vi "configuration UI.vi"() -> ()   [LabVIEW 2013, in "fixed channel editor.lvclass"]
uses:
  fixed channel editor.lvclass
  <vilib>/CEF_TreeControl/Node/NodeRef.ctl
  <vilib>/CEF_TreeControl/Node/NISE_CEF_Node.lvclass
  <vilib>/NI/AMC/Message Queue.ctl
  <vilib>/NI/AMC/Message.ctl
  <vilib>/NI/Tools/Keyed Array/KeyedArray.ctl
  <vilib>/CEF_TreeControl/Node/UserEventRef.ctl
  <vilib>/CEF_TreeControl/Controls/EventCluster.ctl
  <vilib>/NI/Tag Bus Module Framework/root configuration/TBM configuration.lvclass/TBM configuration.ctl
  <vilib>/NI/Tag Bus Module Framework/module configuration/TBM module configuration.lvclass
  <vilib>/NI/Tag Bus Module Framework/channel/TBM channel.lvclass
  <vilib>/NI/Tag Bus/tag/tag descriptor.lvclass/tag descriptor.ctl
  <vilib>/NI/Tag Bus Module Framework/channel/channel classification.ctl
  module/configuration/fixed channel configuration.lvclass
  <vilib>/NI/Tag Bus Module Framework/root configuration/Read instance name.vi
  read fixed channel configuration.vi
  <vilib>/NI/Tag Bus Module Framework/root configuration/create GUID.vi
  <vilib>/NI/Tag Bus Data Framework/Configuration Editor/Classes/Module editor node/Read Module Configuration.vi
  <vilib>/NI/Module Execution Interface/Engine Configuration/engine configuration.lvclass
  <vilib>/NI/Tag Bus/tag/tag descriptor.lvclass
  <vilib>/CEF_TreeControl/NISE_CEF_TreeControl.lvlib
  <vilib>/NI/Tag Bus Data Framework/Configuration Editor/Classes/Engine Parent/Engine Parent Editor Node.lvclass
  <vilib>/NI/Tag Bus Data Framework/Configuration Editor/Classes/Module editor node/module editor node.lvclass
  <vilib>/NI/Tools/Keyed Array/Tools_KeyedArray.lvlib
  <vilib>/NI/AMC/AMC.lvlib
panel:
  in  "Tab Control":enum32{"Channels", "Parameters"}(tab)
  in  "mapwriters":bool
  out "Channel List":string[][](table)
  in  "mapall":bool
  in  "kvp":i32(listbox)
  in  "user event":T1
  in  "main queue":T2
  in  "node ref":T3
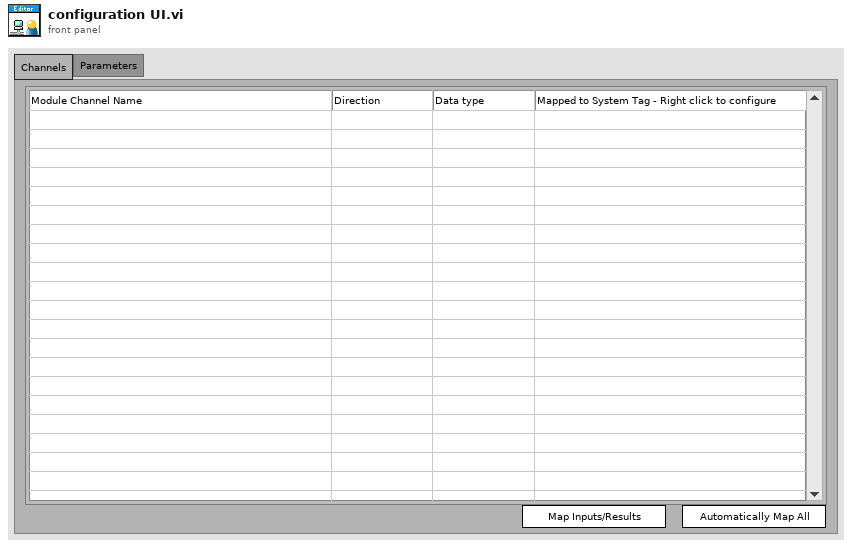
[diagram p1: front panel]
types:
  T1 = typedef "NISE_CEF_Node.lvclass/UserEventRef.ctl" = refnum<user-event>
  T2 = typedef "AMC.lvlib/Message Queue.ctl" = refnum<queue>
  T3 = typedef "NISE_CEF_Node.lvclass/NodeRef.ctl" = refnum<data-value>
  T4 = typedef "NISE_CEF_TreeControl.lvlib/EventCluster.ctl" = cluster{"command":string, "data":string}
  T5 = typedef "LVPoint32TypeDef.ctl" = cluster{"Horizontal":i32, "Vertical":i32}
  T6 = typedef "LVRowAndColumnTypeDef.ctl" = cluster{"Row":i32, "Column":i32}
  T7 = typedef "TBM channel.lvclass/channel classification.ctl" = enum16{"input data", "output data", "processing parameter", "processing result"}
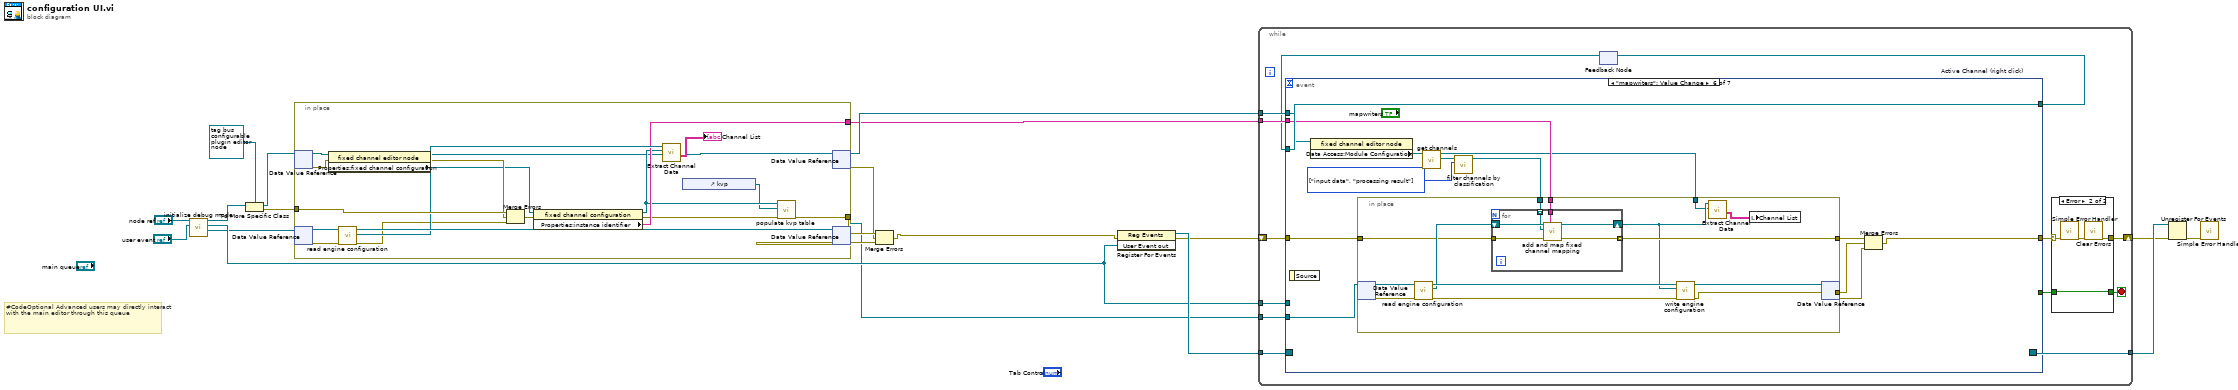
[diagram p0: block diagram]
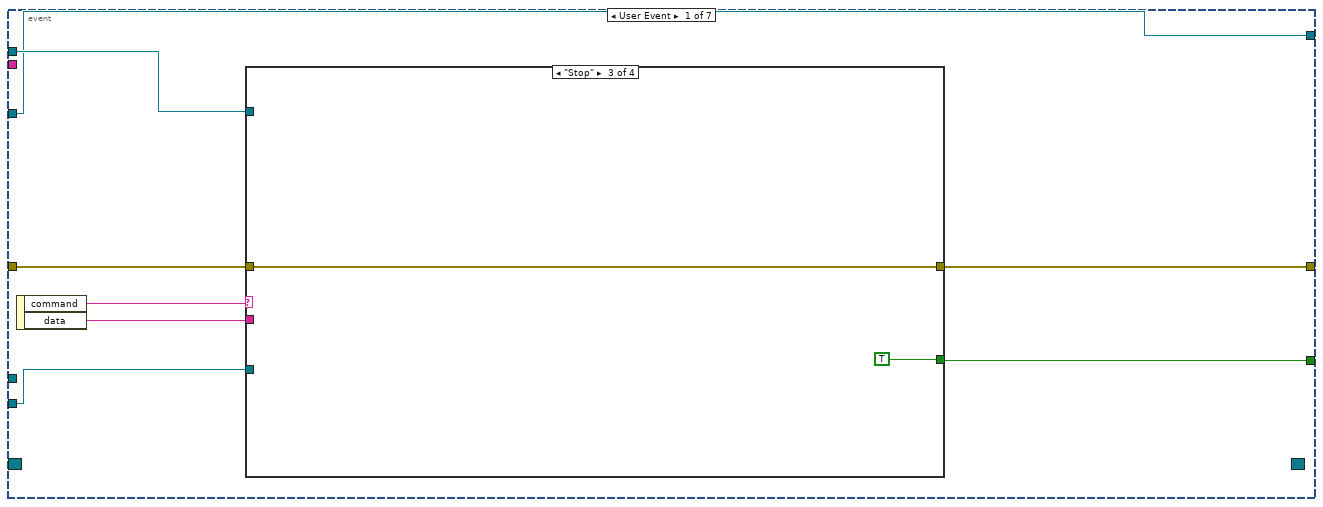
[diagram p3: hidden frame]
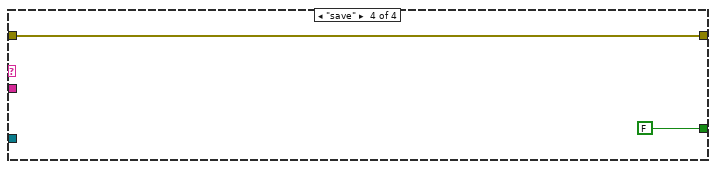
[diagram p6: hidden frame]
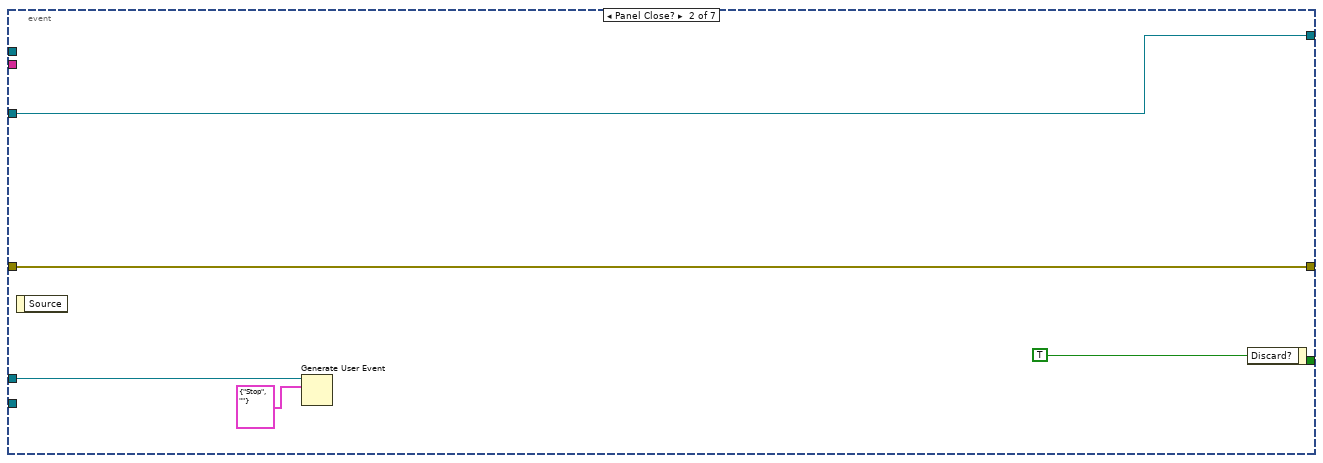
[diagram p7: hidden frame]
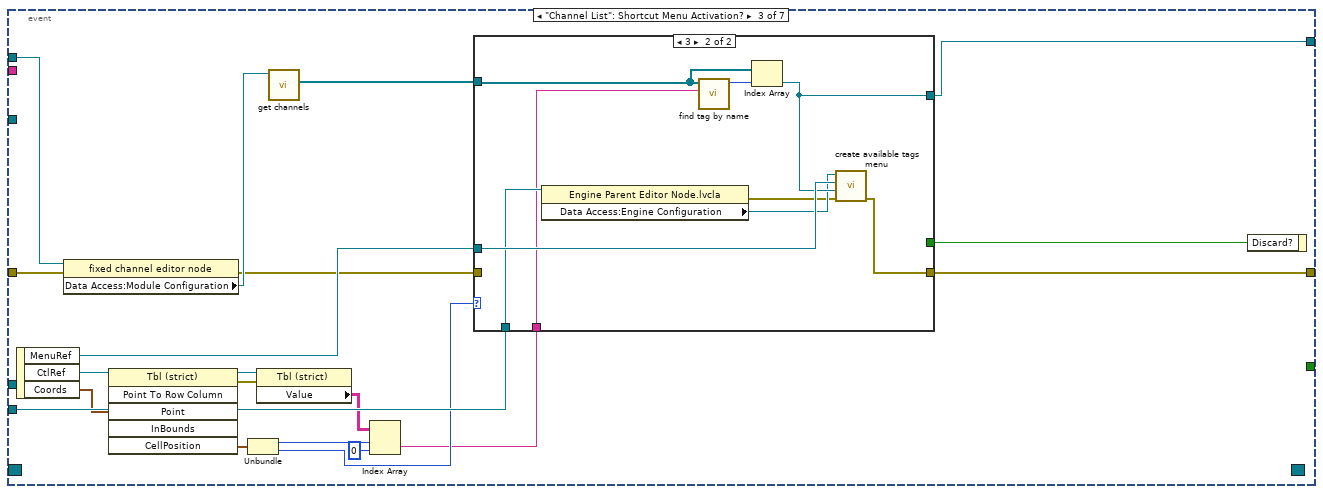
[diagram p8: hidden frame]
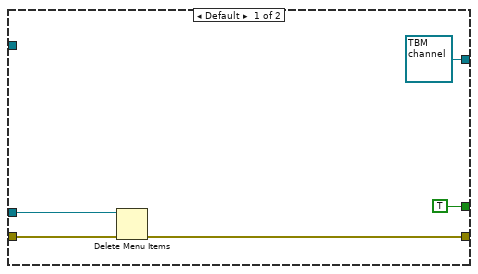
[diagram p9: hidden frame]
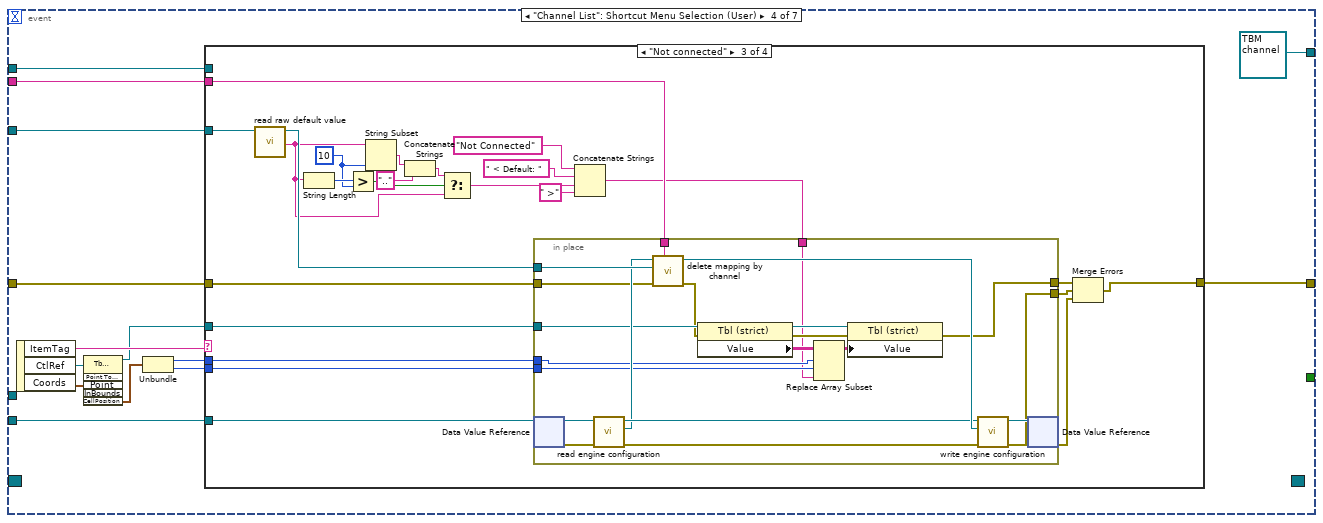
[diagram p10: hidden frame]
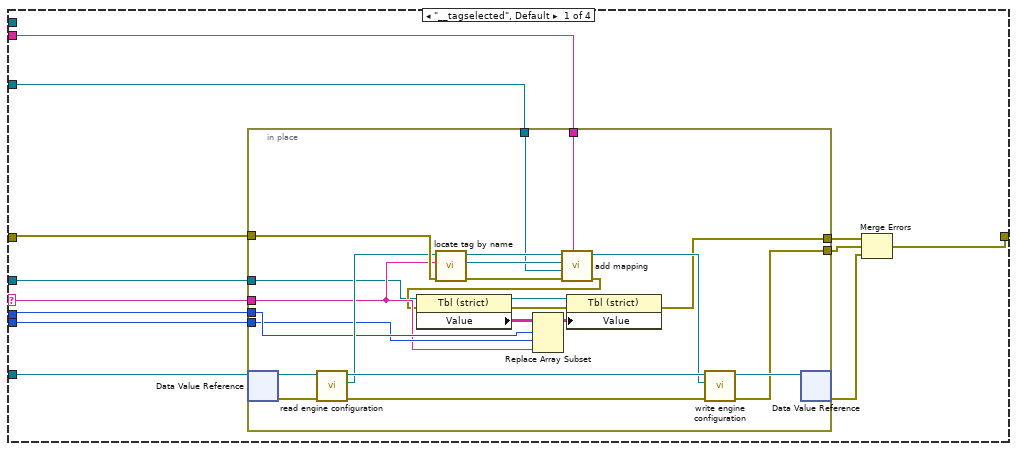
[diagram p11: hidden frame]
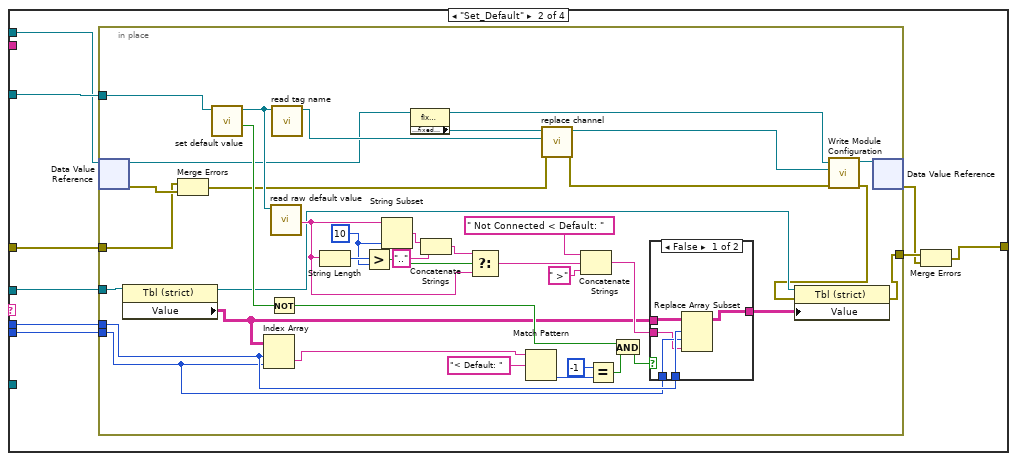
[diagram p12: hidden frame]
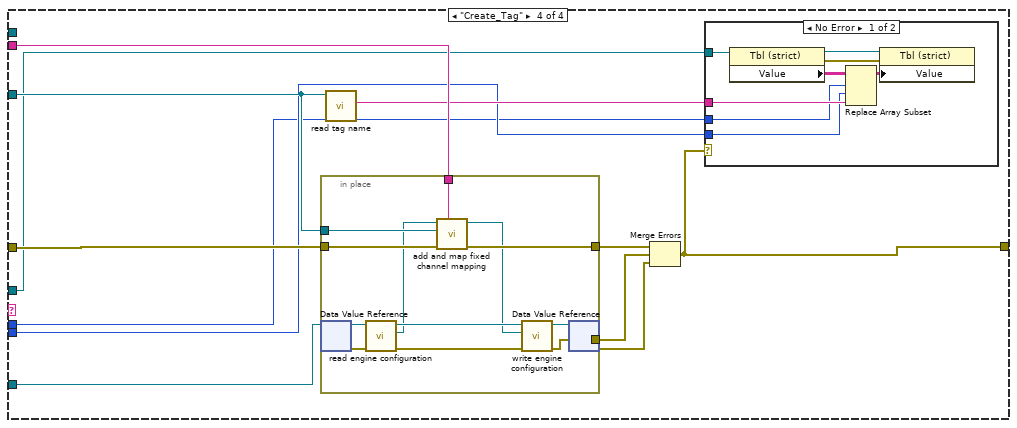
[diagram p14: hidden frame]
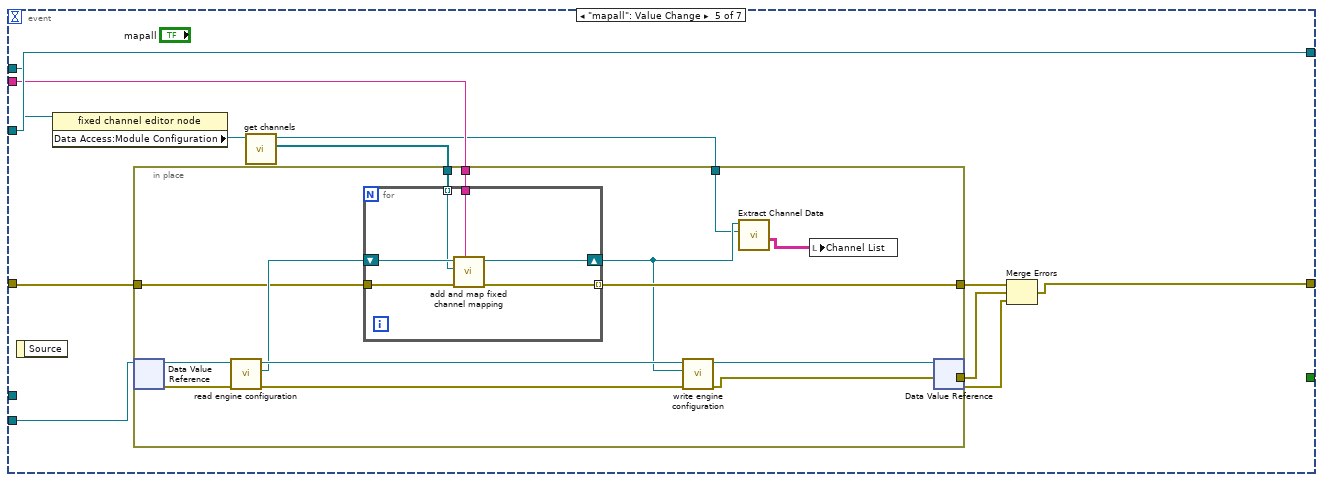
[diagram p16: hidden frame]
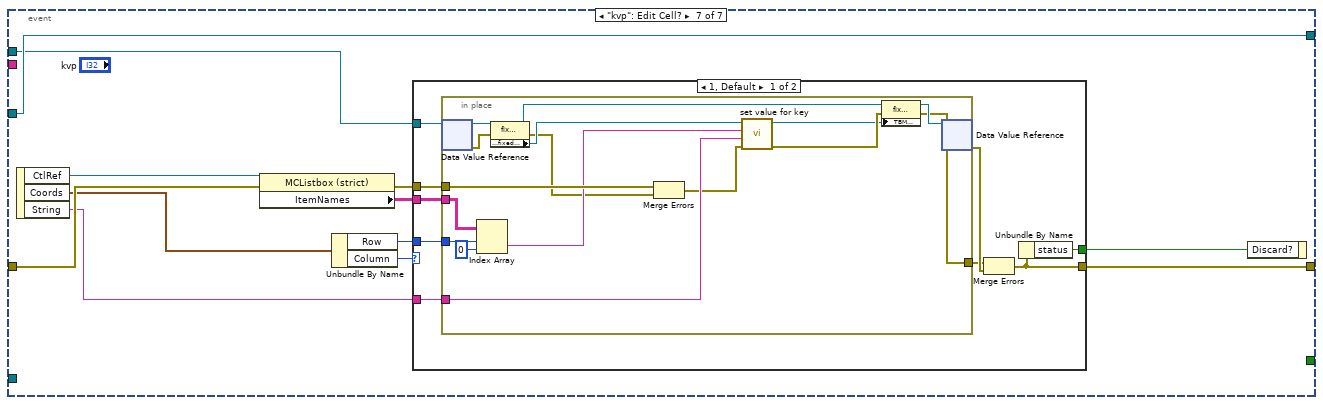
[diagram p17: hidden frame]
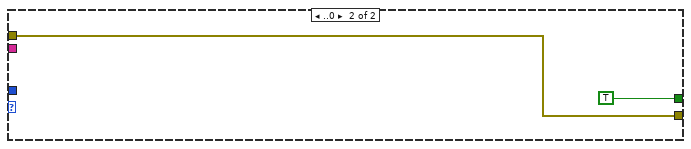
[diagram p18: hidden frame]
diagram:
  # "#CodeOptional Advanced users may directly interact with the main editor through this queue"
  n1 = call "initialize debug mode.vi"("User Event in"="user event", "editor node in"="node ref") -> ("engine"=w4:refnum<data-value>, "User Event out"=w11:T1, "editor node out"=w14:T3)  [unwired: 7 in]
  n2 = To More Specific Class(target class=refnum<data-value> refnum ("data value reference"), reference=w14) -> (specific class reference=w10:refnum<data-value>, error out=w8:errorcluster)  [unwired: 1 in]
  n3 = in-place {
    in-place-border: w8 -> [w38]
    in-place-border: [w26] -> w7
    in-place-border: [w31] -> w2
    n4 = in-place-dvr #1(w10) -> (w35:refnum<class "fixed channel editor.lvclass">, w23:errorcluster)
    n5 = in-place-dvr #2(w4) -> (w37:refnum<class "Engine Parent Editor Node.lvclass">, w29:errorcluster)
    n6 = property class="fixed channel editor node"(reference=w35, error in=w23) -> (reference out=w24:refnum<class "fixed channel editor.lvclass">, error out=w22:errorcluster, "Properties:fixed channel configuration"=w21:refnum<class "fixed channel configuration.lvclass">)
    n7 = call <vilib>:"read engine configuration.vi"("error in"=w29, "Engine Parent Editor Node in"=w37) -> ("error out"=w30:errorcluster, "engine configuration"=w33:refnum<class "engine configuration.lvclass">, "Engine Parent Editor Node out"=w36:refnum<class "Engine Parent Editor Node.lvclass">)  [unwired: 7 in]
    n8 = Merge Errors(w38, w22, w30) -> (w34:errorcluster)
    n9 = property class="fixed channel configuration"(reference=w21, error in=w34) -> (reference out=w28:refnum<class "fixed channel configuration.lvclass">, error out=w27:errorcluster, "Properties:instance identifier"=w31:string)
    n10 = call "Extract Channel Data.vi"("module configuration in"=w28, "Engine Configuration"=w33) -> ("Channel Data"=→"Channel List":string[][])  [unwired: 9 in]
    n11 = control-ref of="kvp"() -> (w25:refnum<vi>)
    n12 = call "populate kvp table.vi"("error in"=w27, "MCListbox Refnum"=w25, "fixed channel configuration in"=w28) -> ("error out"=w26:errorcluster)  [unwired: 8 in]
    n13 = in-place-dvr #1(w24) -> (w9:refnum<data-value>, w5:errorcluster)
    n14 = in-place-dvr #2(w36) -> (w3:refnum<data-value>, w6:errorcluster)
  }
  n15 = Merge Errors(w7, w5, w6) -> (w1:errorcluster)
  n16 = register-events(error in=w1, w11) -> (reference out=w20:refnum<event-registration>, error out=w16:errorcluster)  [unwired: 1 in]
  n17 = while {
    tunnel: w20 -> [w51]
    tunnel: [w50] -> w19
    shift-right: [w46] -> w18
    shift-left: w16 -> [w49]
    tunnel: w2 -> [w45]
    tunnel: w9 -> [w44]
    tunnel: w3 -> [w43]
    tunnel: w11 -> [w40]
    stop <- w47 stop-if-true
    n18 = feedback #3 "Active Channel (right click)"() -> (w41:refnum<class "TBM channel.lvclass">)  [unwired: 1 in]
    n19 = event shown="[5] \"mapwriters\": Value Change" {
      selector: w51 -> [_ _ _ _ _ _ _]
      dyn-events: [_ _ _ _ _ _ _] -> w50
      timeout: _ -> [_ _ _ _ _ _ _]
      tunnel: [w64 _ _ _ _ _ _] -> w39
      tunnel: [w65 w76 w78 w120 w293 w328 w363] -> w48
      tunnel: w49 -> [w59 w76 w96 w121 w297 w331 w367]
      tunnel: w45 -> [_ _ _ w119 w302 w336 _]
      tunnel: w44 -> [w62 _ w93 w117 w296 w330 w359]
      tunnel: w43 -> [w61 _ w94 w118 w298 w332 _]
      tunnel: w41 -> [w58 w75 _ w122 w303 w337 w369]
      tunnel: [w58 w75 w95 refnum<class "TBM channel.lvclass"> refnum ("channel") w303 w337 w369] -> w42
      tunnel: w40 -> [_ w73 _ _ _ _ _]
      event User Event {
        n20 = event-data() -> ("command"=w63:string, "data"=w60:string)  [unwired: 1 in]
        n21 = case shown="\"Stop\"" w63 {
          tunnel: [_ _ TRUE FALSE] -> w64
          tunnel: w61 -> [_ _ _ _]
          tunnel: w59 -> [w66 w67 w68 w70]
          tunnel: [w66 w67 w68 w70] -> w65
          tunnel: w62 -> [_ _ _ _]
          tunnel: w60 -> [_ _ _ _]
          frame Default {
          }
          frame "Refresh" {
          }
          frame "Stop" {
          }
          frame "save" {
          }
        }
      }
      event Panel Close? {
        n22 = event-data() -> ()  [unwired: 1 in, 1 out]
        n23 = Generate User Event(user event=w73, event data cluster=T4 {"command"="Stop", "data"=""} ("event data")) -> ()  [unwired: 2 in, 2 out]
        n24 = event-data("Discard?"=TRUE) -> ()  [unwired: 1 in, 1 out]
      }
      event "Channel List": Shortcut Menu Activation? {
        n25 = event-data() -> ("MenuRef"=w89:refnum<k9>, "CtlRef"=w90:refnum<vi>, "Coords"=w88:T5)  [unwired: 1 in]
        n26 = property class="fixed channel editor node"(reference=w93, error in=w96) -> (error out=w79:errorcluster, "Data Access:Module Configuration"=w92:refnum<class "TBM module configuration.lvclass">)  [unwired: 1 out]
        n27 = invoke class="Tbl (strict)" method="Point To Row Column"(reference=w90, "Point"=w88) -> (reference out=w86:refnum<vi>, error out=w85:errorcluster, "CellPosition"=w87:T6)  [unwired: 4 in, 3 out]
        n28 = Unbundle(w87) -> ("Row"=w83:i32, "Column"=w81:i32)
        n29 = property class="Tbl (strict)"(reference=w86, error in=w85) -> ("Value"=w84:string[][])  [unwired: 2 out]
        n30 = call-dynamic "get channels.vi"("module configuration in"=w92) -> ("channels"=w91:refnum<class "TBM channel.lvclass">[])  [unwired: 9 in, 1 out]
        n31 = Index Array(array=w84, index (row)=w83, index (col)=0 ("disabled index (col)")) -> (element=w80:string)
        n32 = case shown="3" w81 {
          tunnel: w89 -> [w100 w110]
          tunnel: [w98 w102] -> w78
          tunnel: w91 -> [_ w104]
          tunnel: [refnum<class "TBM channel.lvclass"> refnum ("channel") w109] -> w95
          tunnel: w94 -> [_ w107]
          tunnel: w80 -> [_ w105]
          tunnel: w79 -> [w99 _]
          tunnel: [TRUE _] -> w77
          frame Default {
            n33 = Delete Menu Items(6:w99, 9:w100) -> (0:w98:errorcluster)  [unwired: 2 in, 1 out]
          }
          frame 3 {
            n34 = property class="Engine Parent Editor Node.lvcla"(reference=w107) -> (error out=w103:errorcluster, "Data Access:Engine Configuration"=w106:refnum<class "engine configuration.lvclass">)  [unwired: 1 in, 1 out]
            n35 = call <vilib>:"find tag by name.vi"("name"=w105, "tags in"=w104) -> ("index"=w108:i32)  [unwired: 9 in]
            n36 = Index Array(array=w104, index=w108) -> (element=w109:refnum<class "TBM channel.lvclass">)
            n37 = call "create available tags menu.vi"("error in"=w103, "channel to map to"=w109, "MenuRef"=w110, "engine configuration in"=w106) -> ("error out"=w102:errorcluster)  [unwired: 6 in, 1 out]
          }
        }
        n38 = event-data("Discard?"=w77) -> ()  [unwired: 1 in, 1 out]
      }
      event "Channel List": Shortcut Menu Selection (User) {
        n39 = event-data() -> ("ItemTag"=w124:string, "CtlRef"=w116:refnum<vi>, "Coords"=w115:T5)  [unwired: 1 in]
        n40 = invoke class="Tbl (strict)" method="Point To Row Column"(reference=w116, "Point"=w115) -> (reference out=w111:refnum<vi>, "CellPosition"=w114:T6)  [unwired: 4 in, 4 out]
        n41 = Unbundle(w114) -> ("Row"=w113:i32, "Column"=w112:i32)
        n42 = case shown="\"Not connected\"" w124 {
          selector: w124 -> [w134 _ _ _]
          tunnel: w112 -> [w136 w168 w238 w262]
          tunnel: w113 -> [w135 w167 w237 w261]
          tunnel: w122 -> [w132 w169 w233 w265]
          tunnel: [w129 w165 w218 w263] -> w120
          tunnel: w121 -> [w133 w161 w236 w271]
          tunnel: w119 -> [w130 _ w234 w269]
          tunnel: w118 -> [w126 _ w219 w268]
          tunnel: w117 -> [_ w166 _ _]
          tunnel: w111 -> [w125 w162 w215 w260]
          frame "__tagselected", Default {
            n43 = in-place {
              in-place-border: w136 -> [w141]
              in-place-border: w135 -> [w142]
              in-place-border: w134 -> [w140]
              in-place-border: w133 -> [w160]
              in-place-border: w132 -> [w157]
              in-place-border: [w138] -> w131
              in-place-border: w130 -> [w155]
              in-place-border: [w149] -> w127
              in-place-border: w125 -> [w137]
              n44 = in-place-dvr #4(w126) -> (w152:refnum<class "Engine Parent Editor Node.lvclass">, w151:errorcluster)
              n45 = call <vilib>:"read engine configuration.vi"("error in"=w151, "Engine Parent Editor Node in"=w152) -> ("error out"=w153:errorcluster, "engine configuration"=w147:refnum<class "engine configuration.lvclass">, "Engine Parent Editor Node out"=w154:refnum<class "Engine Parent Editor Node.lvclass">)  [unwired: 7 in]
              n46 = call <vilib>:"locate tag by name.vi"("error in"=w160, "tag name"=w140, "engine configuration in"=w147) -> ("error out"=w156:errorcluster, "tag descriptor"=w158:refnum<class "tag descriptor.lvclass">, "engine configuration out"=w159:refnum<class "engine configuration.lvclass">)  [unwired: 6 in]
              n47 = call <vilib>:"add mapping.vi"("owner ID"=w155, "error in"=w156, "channel"=w157, "tag descriptor"=w158, "engine configuration"=w159) -> ("error out"=w139:errorcluster, "engine configuration out"=w148:refnum<class "engine configuration.lvclass">)  [unwired: 5 in]
              n48 = property class="Tbl (strict)"(reference=w137, error in=w139) -> (reference out=w144:refnum<vi>, error out=w145:errorcluster, "Value"=w143:string[][])
              n49 = Replace Array Subset(array=w143, new element=w140, index (row)=w142, index (col)=w141) -> (w146:string[][])
              n50 = property class="Tbl (strict)"(reference=w144, error in=w145, "Value"=w146) -> (error out=w138:errorcluster)  [unwired: 1 out]
              n51 = call <vilib>:"write engine configuration.vi"("error in"=w153, "engine configuration"=w148, "Engine Parent Editor Node in"=w154) -> ("error out"=w149:errorcluster, "Engine Parent Editor Node out"=w150:refnum<class "Engine Parent Editor Node.lvclass">)  [unwired: 7 in]
              n52 = in-place-dvr #4(w150) -> (w128:errorcluster)  [unwired: 1 out]
            }
            n53 = Merge Errors(w131, w127, w128) -> (w129:errorcluster)
          }
          frame "Set_Default" {
            n54 = in-place {
              in-place-border: w169 -> [w208]
              in-place-border: w168 -> [w177]
              in-place-border: w167 -> [w178]
              in-place-border: [w175] -> w164
              in-place-border: w162 -> [w183]
              in-place-border: w161 -> [w170]
              w197 = 10 ("y")
              n55 = in-place-dvr #5(w166) -> (w173:refnum<class "fixed channel editor.lvclass">, w186:errorcluster)
              n56 = property class="Tbl (strict)"(reference=w183) -> (reference out=w181:refnum<vi>, "Value"=w180:string[][])  [unwired: 1 in, 1 out]
              n57 = Merge Errors(w170, w186) -> (w171:errorcluster)
              n58 = call "set default value.vi"("tag"=w208) -> ("cancelled?"=w200:bool, "tag out"=w192:refnum<class "TBM channel.lvclass">)  [unwired: 9 in]
              n59 = Index Array(array=w180, index (row)=w178, index (col)=w177) -> (element=w179:string)
              n60 = Not(x=w200) -> (.not. x?=w189:bool)
              n61 = call <vilib>:"read raw default value.vi"("system tag in"=w192) -> ("raw default"=w193:string)  [unwired: 8 in, 2 out]
              n62 = call <vilib>:"read tag name.vi"("system tag in"=w192) -> ("system tag out"=w184:refnum<class "TBM channel.lvclass">)  [unwired: 8 in, 2 out]
              n63 = String Length(string=w193) -> (length=w199:i32)
              n64 = Greater?(x=w199, y=w197) -> (0:w198:bool)
              n65 = String Subset(string=w193, length (rest)=w197) -> (substring=w195:string)  [unwired: 1 in]
              n66 = property class="fixed channel editor node"(reference=w173) -> (reference out=w172:refnum<class "fixed channel editor.lvclass">, "Properties:fixed channel configuration"=w174:refnum<class "fixed channel configuration.lvclass">)  [unwired: 1 in, 1 out]
              n67 = Concatenate Strings(w195, ".." ("string")) -> (w196:string)
              n68 = Select(t=w196, s=w198, f=w193) -> (s? t:f=w191:string)
              n69 = Match Pattern(string=w179, regular expression="< Default: ") -> (offset past match=w206:i32)  [unwired: 1 in, 3 out]
              n70 = call "replace channel.vi"("error in"=w171, "channel"=w184, "fixed module parent implementation configuration in"=w174) -> ("error out"=w185:errorcluster, "fixed module parent implementation configuration out"=w187:refnum<class "fixed channel configuration.lvclass">)  [unwired: 7 in]
              n71 = Concatenate Strings(" Not Connected < Default: " ("string"), w191, " >" ("string")) -> (w190:string)
              n72 = Equal?(x=-1, y=w206) -> (x = y?=w204:bool)
              n73 = And(x=w189, y=w204) -> (x .and. y?=w201:bool)
              n74 = case shown="False" w201 {
                tunnel: w190 -> [w209 _]
                tunnel: w180 -> [w213 w214]
                tunnel: [w212 w214] -> w182
                tunnel: w178 -> [w211 _]
                tunnel: w177 -> [w210 _]
                frame False {
                  n75 = Replace Array Subset(array=w213, new element=w209, index (row)=w211, index (col)=w210) -> (w212:string[][])
                }
                frame True {
                }
              }
              n76 = call <vilib>:"Write Module Configuration.vi"("error in"=w185, "module configuration"=w187, "Module Editor Node in"=w172) -> ("error out"=w176:errorcluster, "Module Editor Node out"=w188:refnum<class "fixed channel editor.lvclass">)  [unwired: 7 in]
              n77 = property class="Tbl (strict)"(reference=w181, error in=w176, "Value"=w182) -> (error out=w175:errorcluster)  [unwired: 1 out]
              n78 = in-place-dvr #5(w188) -> (w163:errorcluster)  [unwired: 1 out]
            }
            n79 = Merge Errors(w164, w163) -> (w165:errorcluster)
          }
          frame "Not connected" {
            w226 = 10 ("y")
            n80 = call <vilib>:"read raw default value.vi"("system tag in"=w233) -> ("raw default"=w222:string, "system tag out"=w232:refnum<class "TBM channel.lvclass">)  [unwired: 8 in, 1 out]
            n81 = String Length(string=w222) -> (length=w228:i32)
            n82 = Greater?(x=w228, y=w226) -> (0:w227:bool)
            n83 = String Subset(string=w222, length (rest)=w226) -> (substring=w224:string)  [unwired: 1 in]
            n84 = Concatenate Strings(w224, ".." ("string")) -> (w225:string)
            n85 = Select(t=w225, s=w227, f=w222) -> (s? t:f=w221:string)
            n86 = Concatenate Strings("Not Connected" ("string"), " < Default: " ("string"), w221, " >" ("string")) -> (w231:string)
            n87 = in-place {
              in-place-border: w238 -> [w244]
              in-place-border: w237 -> [w245]
              in-place-border: w236 -> [w241]
              in-place-border: [w239] -> w235
              in-place-border: w234 -> [w259]
              in-place-border: w232 -> [w258]
              in-place-border: w231 -> [w242]
              in-place-border: [w253] -> w216
              in-place-border: w215 -> [w243]
              n88 = in-place-dvr #6(w219) -> (w257:refnum<class "Engine Parent Editor Node.lvclass">, w256:errorcluster)
              n89 = call <vilib>:"read engine configuration.vi"("error in"=w256, "Engine Parent Editor Node in"=w257) -> ("error out"=w254:errorcluster, "engine configuration"=w250:refnum<class "engine configuration.lvclass">, "Engine Parent Editor Node out"=w251:refnum<class "Engine Parent Editor Node.lvclass">)  [unwired: 7 in]
              n90 = call <vilib>:"delete mapping by channel.vi"("owner ID"=w259, "error in"=w241, "channel"=w258, "engine configuration in"=w250) -> ("error out"=w240:errorcluster, "engine configuration out"=w252:refnum<class "engine configuration.lvclass">)  [unwired: 6 in]
              n91 = property class="Tbl (strict)"(reference=w243, error in=w240) -> (reference out=w247:refnum<vi>, error out=w248:errorcluster, "Value"=w246:string[][])
              n92 = Replace Array Subset(array=w246, new element=w242, index (row)=w245, index (col)=w244) -> (w249:string[][])
              n93 = property class="Tbl (strict)"(reference=w247, error in=w248, "Value"=w249) -> (error out=w239:errorcluster)  [unwired: 1 out]
              n94 = call <vilib>:"write engine configuration.vi"("error in"=w254, "engine configuration"=w252, "Engine Parent Editor Node in"=w251) -> ("error out"=w253:errorcluster, "Engine Parent Editor Node out"=w255:refnum<class "Engine Parent Editor Node.lvclass">)  [unwired: 7 in]
              n95 = in-place-dvr #6(w255) -> (w217:errorcluster)  [unwired: 1 out]
            }
            n96 = Merge Errors(w235, w216, w217) -> (w218:errorcluster)
          }
          frame "Create_Tag" {
            n97 = in-place {
              in-place-border: w271 -> [w291]
              in-place-border: [w290] -> w270
              in-place-border: w269 -> [w289]
              in-place-border: w265 -> [w288]
              in-place-border: [w284] -> w266
              n98 = in-place-dvr #7(w268) -> (w286:refnum<class "Engine Parent Editor Node.lvclass">, w287:errorcluster)
              n99 = call <vilib>:"read engine configuration.vi"("error in"=w287, "Engine Parent Editor Node in"=w286) -> ("error out"=w283:errorcluster, "engine configuration"=w281:refnum<class "engine configuration.lvclass">, "Engine Parent Editor Node out"=w282:refnum<class "Engine Parent Editor Node.lvclass">)  [unwired: 7 in]
              n100 = call <vilib>:"add and map fixed channel mapping.vi"("module instance"=w289, "error in"=w291, "fixed channel"=w288, "engine configuration in"=w281) -> ("error out"=w290:errorcluster, "engine configuration out"=w280:refnum<class "engine configuration.lvclass">)  [unwired: 6 in]
              n101 = call <vilib>:"write engine configuration.vi"("error in"=w283, "engine configuration"=w280, "Engine Parent Editor Node in"=w282) -> ("error out"=w284:errorcluster, "Engine Parent Editor Node out"=w285:refnum<class "Engine Parent Editor Node.lvclass">)  [unwired: 7 in]
              n102 = in-place-dvr #7(w285) -> (w267:errorcluster)  [unwired: 1 out]
            }
            n103 = call <vilib>:"read tag name.vi"("system tag in"=w265) -> ("name"=w264:string)  [unwired: 8 in, 2 out]
            n104 = Merge Errors(w270, w266, w267) -> (w263:errorcluster)
            n105 = case shown="No Error" w263 {
              tunnel: w264 -> [w275 _]
              tunnel: w262 -> [w274 _]
              tunnel: w261 -> [w273 _]
              tunnel: w260 -> [w272 _]
              frame No Error {
                n106 = property class="Tbl (strict)"(reference=w272) -> (reference out=w277:refnum<vi>, error out=w278:errorcluster, "Value"=w276:string[][])  [unwired: 1 in]
                n107 = Replace Array Subset(array=w276, new element=w275, index (row)=w273, index (col)=w274) -> (w279:string[][])
                n108 = property class="Tbl (strict)"(reference=w277, error in=w278, "Value"=w279) -> ()  [unwired: 2 out]
              }
              frame Error {
              }
            }
          }
        }
      }
      event "mapall": Value Change {
        n109 = event-data() -> ()  [unwired: 1 in, 1 out]
        n110 = property class="fixed channel editor node"(reference=w296) -> ("Data Access:Module Configuration"=w295:refnum<class "TBM module configuration.lvclass">)  [unwired: 1 in, 2 out]
        n111 = call-dynamic "get channels.vi"("module configuration in"=w295) -> ("channels"=w294:refnum<class "TBM channel.lvclass">[], "module configuration out"=w292:refnum<class "TBM module configuration.lvclass">)  [unwired: 9 in]
        n112 = in-place {
          in-place-border: [w317] -> w301
          in-place-border: [w313] -> w300
          in-place-border: w302 -> [w309]
          in-place-border: w297 -> [w308]
          in-place-border: w294 -> [w307]
          in-place-border: w292 -> [w304]
          n113 = in-place-dvr #8(w298) -> (w315:refnum<class "Engine Parent Editor Node.lvclass">, w316:errorcluster)
          n114 = call <vilib>:"read engine configuration.vi"("error in"=w316, "Engine Parent Editor Node in"=w315) -> ("error out"=w312:errorcluster, "engine configuration"=w310:refnum<class "engine configuration.lvclass">, "Engine Parent Editor Node out"=w311:refnum<class "Engine Parent Editor Node.lvclass">)  [unwired: 7 in]
          n115 = for {
            tunnel: [w323] -> w317 mode=indexing
            tunnel: w309 -> [w320]
            tunnel: w308 -> [w319]
            shift-right: [w321] -> w305
            shift-left: w310 -> [w322]
            tunnel: w307 -> [w318] mode=indexing
            n116 = call <vilib>:"add and map fixed channel mapping.vi"("module instance"=w320, "error in"=w319, "fixed channel"=w318, "engine configuration in"=w322) -> ("error out"=w323:errorcluster, "engine configuration out"=w321:refnum<class "engine configuration.lvclass">)  [unwired: 6 in]
          }
          n117 = call <vilib>:"write engine configuration.vi"("error in"=w312, "engine configuration"=w305, "Engine Parent Editor Node in"=w311) -> ("error out"=w313:errorcluster, "Engine Parent Editor Node out"=w314:refnum<class "Engine Parent Editor Node.lvclass">)  [unwired: 7 in]
          n118 = call "Extract Channel Data.vi"("module configuration in"=w304, "Engine Configuration"=w305) -> ("Channel Data"=w306:string[][])  [unwired: 9 in]
          n119 = local write "Channel List"(w306) -> ()
          n120 = in-place-dvr #8(w314) -> (w299:errorcluster)  [unwired: 1 out]
        }
        n121 = Merge Errors(w301, w300, w299) -> (w293:errorcluster)
      }
      event "mapwriters": Value Change {
        w326 = T7[] [enum."input data", enum."processing result"] items=["input data", "output data", "processing parameter", "processing result"] ("allowed classifications")
        n122 = event-data() -> ()  [unwired: 1 in, 1 out]
        n123 = property class="fixed channel editor node"(reference=w330) -> ("Data Access:Module Configuration"=w329:refnum<class "TBM module configuration.lvclass">)  [unwired: 1 in, 2 out]
        n124 = call-dynamic "get channels.vi"("module configuration in"=w329) -> ("channels"=w325:refnum<class "TBM channel.lvclass">[], "module configuration out"=w327:refnum<class "TBM module configuration.lvclass">)  [unwired: 9 in]
        n125 = call <vilib>:"filter channels by classification.vi"("allowed classifications"=w326, "channels in"=w325) -> ("channels out"=w324:refnum<class "TBM channel.lvclass">[])  [unwired: 9 in]
        n126 = in-place {
          in-place-border: [w351] -> w335
          in-place-border: [w347] -> w334
          in-place-border: w336 -> [w343]
          in-place-border: w331 -> [w342]
          in-place-border: w324 -> [w341]
          in-place-border: w327 -> [w338]
          n127 = in-place-dvr #9(w332) -> (w349:refnum<class "Engine Parent Editor Node.lvclass">, w350:errorcluster)
          n128 = call <vilib>:"read engine configuration.vi"("error in"=w350, "Engine Parent Editor Node in"=w349) -> ("error out"=w346:errorcluster, "engine configuration"=w344:refnum<class "engine configuration.lvclass">, "Engine Parent Editor Node out"=w345:refnum<class "Engine Parent Editor Node.lvclass">)  [unwired: 7 in]
          n129 = for {
            tunnel: [w357] -> w351 mode=indexing
            tunnel: w343 -> [w354]
            tunnel: w342 -> [w353]
            shift-right: [w355] -> w339
            shift-left: w344 -> [w356]
            tunnel: w341 -> [w352] mode=indexing
            n130 = call <vilib>:"add and map fixed channel mapping.vi"("module instance"=w354, "error in"=w353, "fixed channel"=w352, "engine configuration in"=w356) -> ("error out"=w357:errorcluster, "engine configuration out"=w355:refnum<class "engine configuration.lvclass">)  [unwired: 6 in]
          }
          n131 = call <vilib>:"write engine configuration.vi"("error in"=w346, "engine configuration"=w339, "Engine Parent Editor Node in"=w345) -> ("error out"=w347:errorcluster, "Engine Parent Editor Node out"=w348:refnum<class "Engine Parent Editor Node.lvclass">)  [unwired: 7 in]
          n132 = call "Extract Channel Data.vi"("module configuration in"=w338, "Engine Configuration"=w339) -> ("Channel Data"=w340:string[][])  [unwired: 9 in]
          n133 = local write "Channel List"(w340) -> ()
          n134 = in-place-dvr #9(w348) -> (w333:errorcluster)  [unwired: 1 out]
        }
        n135 = Merge Errors(w335, w334, w333) -> (w328:errorcluster)
      }
      event "kvp": Edit Cell? {
        n136 = event-data() -> ("CtlRef"=w368:refnum<vi>, "Coords"=w358:T6, "String"=w360:string)  [unwired: 1 in]
        n137 = property class="MCListbox (strict)"(reference=w368, error in=w367) -> (error out=w364:errorcluster, "ItemNames"=w362:string[][])  [unwired: 1 out]
        n138 = Unbundle By Name(w358) -> ("Row"=w361:i32, "Column"=w366:i32)
        n139 = case shown="1, Default" w366 {
          tunnel: [w374 TRUE] -> w365
          tunnel: w364 -> [w377 w395]
          tunnel: [w375 w395] -> w363
          tunnel: w362 -> [w373 _]
          tunnel: w361 -> [w372 _]
          tunnel: w360 -> [w371 _]
          tunnel: w359 -> [w378 _]
          frame 1, Default {
            n140 = in-place {
              in-place-border: w377 -> [w394]
              in-place-border: w373 -> [w393]
              in-place-border: w372 -> [w391]
              in-place-border: w371 -> [w389]
              in-place-border: [w379] -> w370
              n141 = in-place-dvr #10(w378) -> (w387:refnum<class "fixed channel editor.lvclass">, w385:errorcluster)
              n142 = Index Array(array=w393, index (row)=w391, index (col)=0 ("disabled index (col)")) -> (element=w390:string)
              n143 = property class="fixed channel editor node"(reference=w387, error in=w385) -> (reference out=w382:refnum<class "fixed channel editor.lvclass">, error out=w384:errorcluster, "Properties:fixed channel configuration"=w386:refnum<class "fixed channel configuration.lvclass">)
              n144 = Merge Errors(w394, w384) -> (w388:errorcluster)
              n145 = call-dynamic "set value for key.vi"("error in"=w388, "value"=w389, "key"=w390, "fixed channel configuration in"=w386) -> ("error out"=w383:errorcluster, "fixed channel configuration out"=w380:refnum<class "fixed channel configuration.lvclass">)  [unwired: 6 in]
              n146 = property class="fixed channel editor node"(reference=w382, error in=w383, "TBM Configuration"=w380) -> (reference out=w381:refnum<class "fixed channel editor.lvclass">, error out=w379:errorcluster)
              n147 = in-place-dvr #10(w381) -> (w376:errorcluster)  [unwired: 1 out]
            }
            n148 = Merge Errors(w370, w376) -> (w375:errorcluster)
            n149 = Unbundle By Name(w375) -> ("status"=w374:bool)
          }
          frame ..0 {
          }
        }
        n150 = event-data("Discard?"=w365) -> ()  [unwired: 1 in, 1 out]
      }
    }
    n151 = feedback-in #3(w42) -> ()
    n152 = case shown="Error" w48 {
      selector: w48 -> [w52 w55]
      tunnel: [w53 w57] -> w47
      tunnel: w39 -> [w53 w57]
      tunnel: [w52 w56] -> w46
      frame No Error {
      }
      frame Error {
        n153 = call <vilib>:"Simple Error Handler.vi"("error in (no error)"=w55) -> ("error out"=w54:errorcluster)  [unwired: 4 in, 4 out]
        n154 = call <vilib>:"Clear Errors.vi"("error in (no error)"=w54) -> ("error out"=w56:errorcluster)  [unwired: 6 in]
      }
    }
  }
  n155 = Unregister For Events(event registration refnum=w19, error in=w18) -> (error out=w15:errorcluster)
  n156 = call <vilib>:"Simple Error Handler.vi"("error in (no error)"=w15) -> ()  [unwired: 4 in, 5 out]
